vi "Log.vi"(9 "LogLevel":i32, 10 "logstring":string, 11 "index":u16) -> (2 "logstring out":string, 3 "function return":i32)   [LabVIEW 2025, in "ExtremelyEpicImagerIPC2.lvlib"]
doc: "IMAGERIPC_API HRESULT WINAPI Log(WORD index, char *logstring, int LogLevel);"
uses:
  ExtremelyEpicImagerIPC2.lvlib
  ImagerIPC2.dll
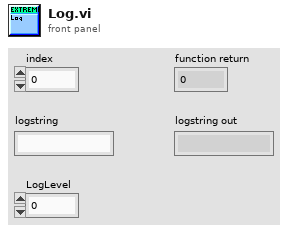
[diagram p1: front panel]
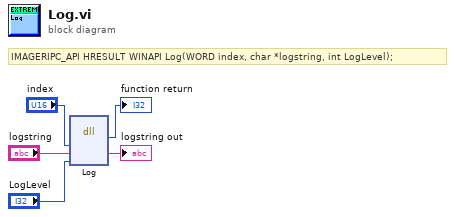
[diagram p0: block diagram]
diagram:
  # "IMAGERIPC_API HRESULT WINAPI Log(WORD index, char *logstring, int LogLevel);"
  n1 = dll-call lib="C:/Users/mayhe/OneDrive/Documents/GitHub/In-situ-monitoring-of-powder-bed-fusion-additive-manufacturing/system_development/Orichalcum/v0.2/Software_design/thermal-camera/VI/Connect SDK/ImagerIPC2.*" fn="Log"("index"="index", "logstring"="logstring", "LogLevel"="LogLevel") -> (→"function return":i32, "logstring"=→"logstring out":string)  [unwired: 5 in, 2 out]
